vi "IMMU - Standalone Main.vi"() -> ()   [LabVIEW 2021]
uses:
  Lab 5/Lab 5 Code/Heading_TDef.ctl
  <vilib>/Platform/TimedLoop/XDataNode/timing_clust.ctl
  <vilib>/Platform/TimedLoop/XDataNode/nitl_modes.ctl
  <vilib>/Platform/TimedLoop/XDataNode/wakeup.ctl
  <vilib>/platform/TimedLoop/XDataNode/XDataNode.xnode
  <vilib>/myRIO/Express VI/Onboard IO/I2C/I2C Express VI.xnode
  <vilib>/myRIO/Instrument Drivers/Onboard IO/I2C/vis/Configure.vi
  <vilib>/myRIO/Instrument Drivers/Onboard IO/I2C/I2C.lvlib
  <vilib>/myRIO/Instrument Drivers/Onboard IO/I2C/typedefs/I2C Transfer Rate.ctl
  <vilib>/myRIO/Instrument Drivers/Onboard IO/I2C/typedefs/I2C User Configuration.ctl
  <vilib>/myRIO/Instrument Drivers/Onboard IO/I2C/typedefs/I2C Configuration.ctl
  <vilib>/myRIO/Common/Instrument Driver Framework/myRIO v1.0/I2C/typedefs/I2C Channels Enum.ctl
  <vilib>/myRIO/Common/Instrument Driver Framework/Utilities/typedefs/Generic FPGA Reference.ctl
  <vilib>/myRIO/Common/Instrument Driver Framework/Utilities/typedefs/myRIO v1.0 Reference.ctl
  <vilib>/myRIO/Common/Instrument Driver Framework/Utilities/typedefs/Hardware Version Enum.ctl
  <vilib>/myRIO/Common/Instrument Driver Framework/Utilities/typedefs/myRIO Generic Hardware Reference.ctl
  <vilib>/myRIO/Instrument Drivers/Onboard IO/I2C/typedefs/I2C Reference.ctl
  <vilib>/myRIO/Instrument Drivers/Onboard IO/I2C/vis/myRIO I2C Open.xnode
  <vilib>/myRIO/Common/Instrument Driver Framework/Utilities/vis/Is FPGA Ref Available.vi
  <vilib>/myRIO/Common/Instrument Driver Framework/myRIO v1.0/I2C/vis/myRIO v1.1 Open I2C.vi
  <vilib>/userDefined/High Color/nirio_resource_hc.ctl
  <vilib>/myRIO/Instrument Drivers/Onboard IO/I2C/vis/Write.vi
  <vilib>/Platform/TimedLoop/XDataNode/XDNodeRunTimeDep.lvlib
panel:
  out "Output Offset Array (int)":i16[](array[numeric])
  out "Mag Flux (uT)":T1(graph)
  out "Heading Output (Str)":T2
  out "Heading":dbl
  in  "Reset Gyro":bool
  out "Acceleration (g)":T3(graph)
  out "Velocity":T1(graph)
  out "Rotation":T3(graph)
  out "Acceleration (ms^2)":dbl[](array[numeric])
  out "error out":errorcluster
  out "Velocity Cluster Out":cluster{i16, i16, i16}
  out "Rotation Cluster Out":T4
  in  "stop":bool
  in  "error in (no error)":errorcluster
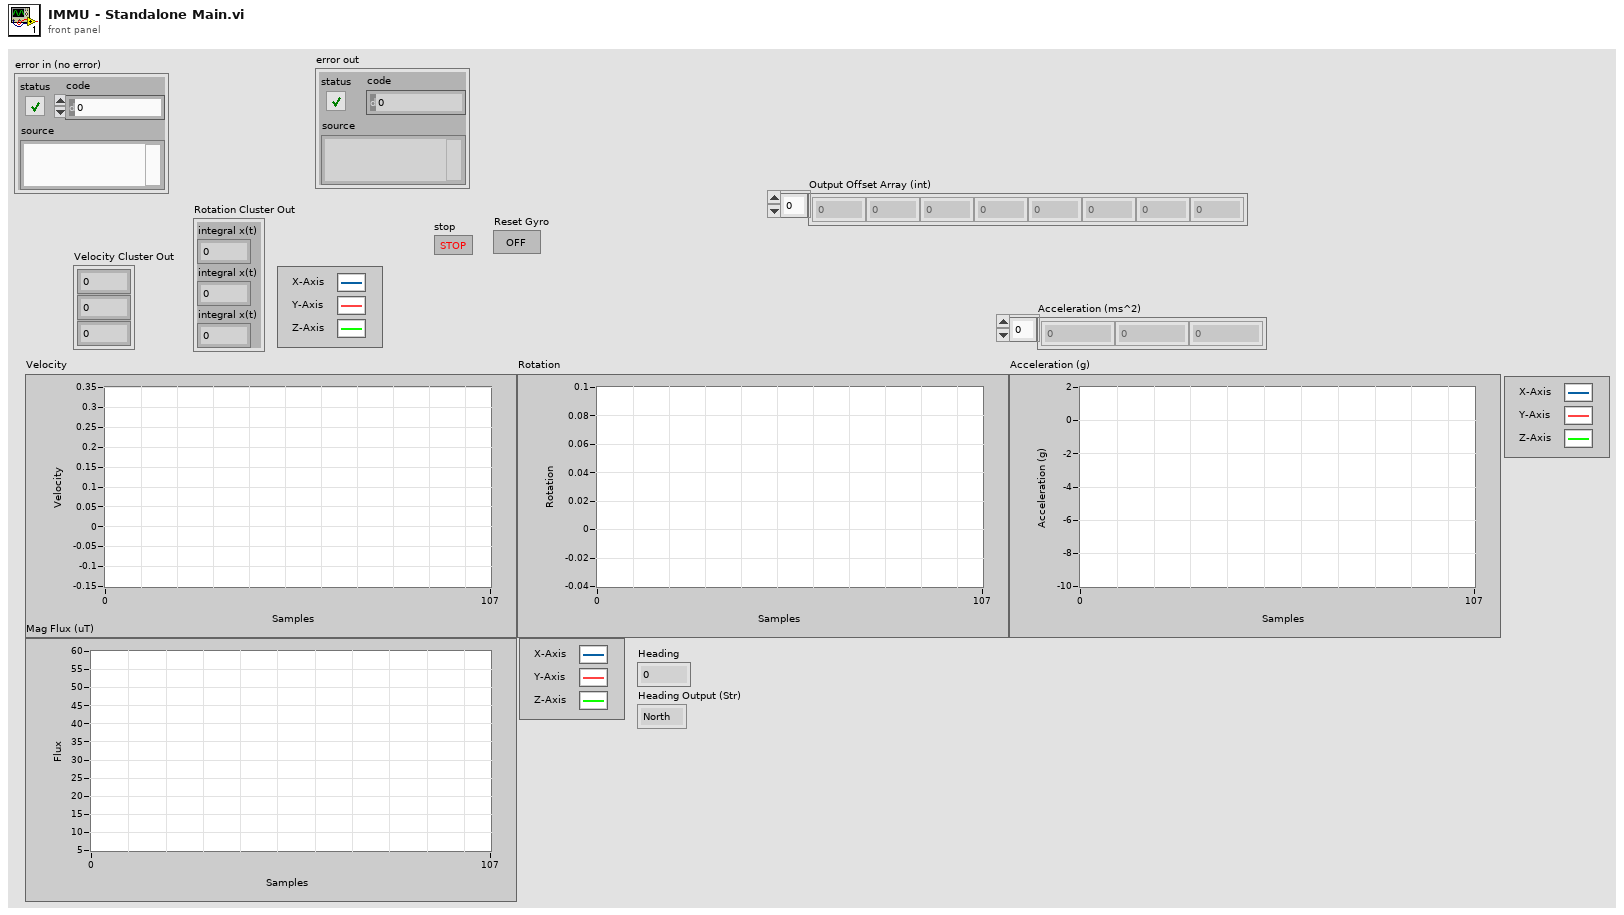
[diagram p1: front panel]
types:
  T1 = cluster{"Velocity":dbl, "Velocity":dbl, "Velocity":dbl}
  T2 = typedef "Heading_TDef.ctl" = enum16{"North ", "North East", "East", "Southeast", "South", "Southwest", "West", "Northwest"}
  T3 = cluster{"X-Axis":dbl, "Y-Axis":dbl, "Z-Axis":dbl}
  T4 = cluster{"integral x(t)":dbl, "integral x(t)":dbl, "integral x(t)":dbl}
  T5 = typedef "I2C.lvlib/I2C Reference.ctl" = cluster{"myRIO Reference":T6, "I2C Channels Enum":T10, "I2C Configuration":T11}
  T6 = typedef "myRIO Generic Hardware Reference.ctl" = cluster{"myRIO Model":T7, "myRIO Hardware Reference":T8}
  T7 = typedef "Hardware Version Enum.ctl" = enum16{"Unknown", "myRIO-1900", "myRIO-1950", "roboRIO", "NI ELVIS RIO CM", "ELVIS III"}
  T8 = typedef "myRIO v1.0 Reference.ctl" = cluster{"Generic FPGA Reference":T9, "Allow multiple opens":bool}
  T9 = typedef "Generic FPGA Reference.ctl" = refnum<k20>
  T10 = typedef "I2C Channels Enum.ctl" = enum16{"Not Connected", "A/I2C", "B/I2C", "I2C/I2C"}
  T11 = typedef "I2C.lvlib/I2C Configuration.ctl" = cluster{"I2C Transfer Rate":T12}
  T12 = typedef "I2C.lvlib/I2C Transfer Rate.ctl" = enum16{"Standard mode (100 kbps)", "Fast mode (400 kbps)"}
  T13 = typedef "I2C.lvlib/I2C User Configuration.ctl" = cluster{"I2C Transfer Rate":T12}
  T14 = typedef "nirio_resource_hc.ctl" = tag
  T15 = typedef "XDNodeRunTimeDep.lvlib/timing_clust.ctl" = cluster{"Expected End [f-1]":u64, "Actual End [f-1]":u64, "Finished Late? [f-1]":bool, "Expected End [i-1]":u64, "Actual End [i-1]":u64, "Finished Late? [i-1]":bool, "Expected Start [i]":u64, "Actual Start [i]":u64, "Expected Start [f]":u64, "Actual Start [f]":u64, "Source Name":string, "Structure Name":string, "Period":i64, "Deadline":i64, "Offset":i64, "Start":i64, "Priority":i32, "Timeout":i32, "Mode":T16, "Wakeup Reason":T17, "Error":errorcluster, "Source Type":string, "Secondary Source Type":string, "Global End Time":u64, "Global Start Time":u64, "Frame Duration":u64, "Iteration Duration":u64, "Assigned CPU":i32, "I/O Scan Engine Mode":u32}
  T16 = typedef "XDNodeRunTimeDep.lvlib/nitl_modes.ctl" = enum32{"No Change", "Process missed periods, maintain original phase", "Discard missed periods, maintain original phase", "Process missed periods, ignore original phase", "Discard missed periods, ignore original phase"}
  T17 = typedef "XDNodeRunTimeDep.lvlib/wakeup.ctl" = enum32{"Normal", "Aborted", "Asynchronous wakeup", "Timing source error", "Timed loop error", "Timeout"}
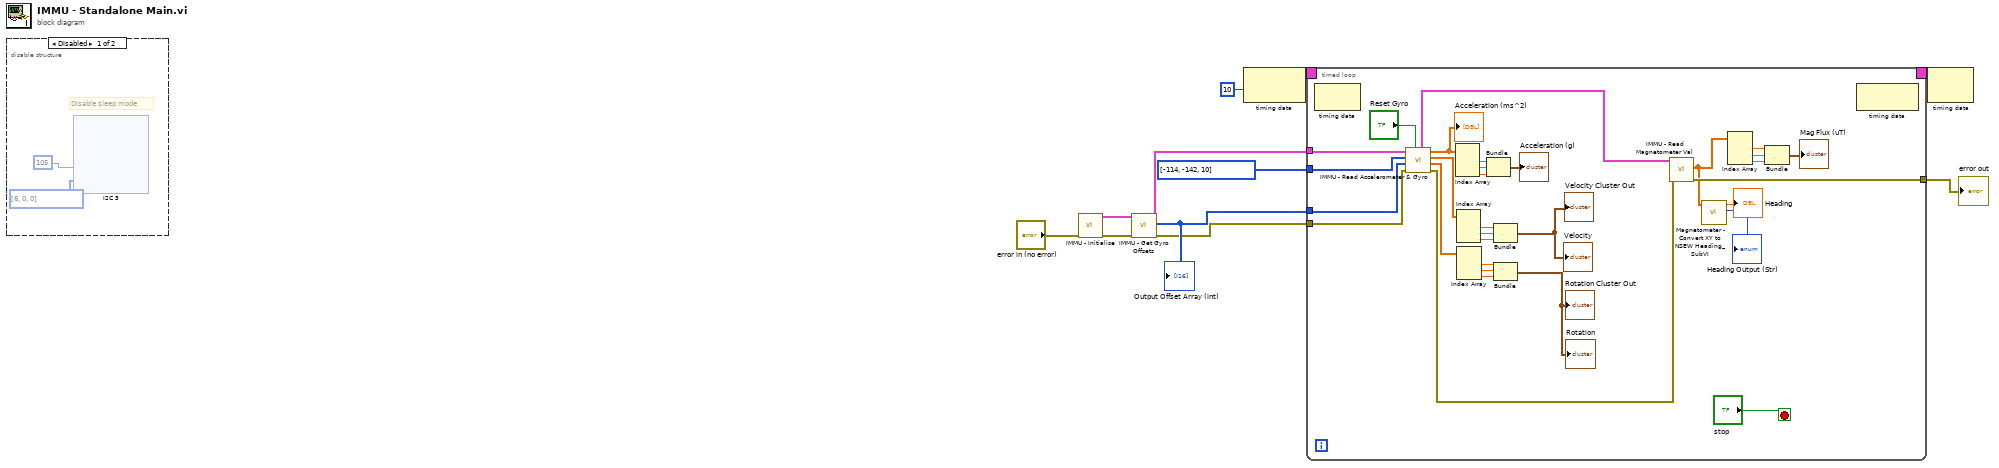
[diagram p0: block diagram]
diagram:
  n1 = disable-structure shown="Disabled" {
    frame Disabled {
      # "Disable sleep mode"
      n2 = xnode "I2C 3"("Slave Address (7-bit)"=u8 105, "Bytes to Write"=u8[] [6, 0, 0]) -> ()  [unwired: 1 in, 1 out]
    }
    frame Enabled {
    }
  }
  n3 = call "IMMU - Initialise.vi"("error in (no error)"="error in (no error)") -> ("error out"=w7:errorcluster, "I2C Ref Out"=w6:T5)  [unwired: 9 in]
  n4 = call "IMMU - Get Gyro Offsets.vi"("error in (no error)"=w7, "I2C Ref In"=w6) -> ("error out"=w2:errorcluster, "Output Offset Array (int)"=w5:i16[], "I2C Ref Out"=w3:T5)  [unwired: 7 in]
  "Output Offset Array (int)" <- w5
  n5 = node-c288(i64 10 ("Period")) -> (w11:T15)
  n6 = timed-loop {
    timing: w11 -> [_]
    timing-out: [_] -> w10
    tunnel: w3 -> [w69]
    tunnel: w2 -> [w68]
    tunnel: w5 -> [w53]
    tunnel: [w60] -> w4
    tunnel: i16[] [-114, -142, 10] ("Accel Offset Array In") -> [w52]
    stop <- "stop" stop-if-true
    n7 = node-c288() -> ()  [unwired: 1 in, 1 out]
    n8 = call "IMMU - Read Accelerometer & Gyro.vi"("Reset Gyro"="Reset Gyro", "error in (no error)"=w68, "Gyro Offset Array In"=w53, "Accel Offset Array In"=w52, "I2C Ref In"=w69) -> ("error out"=w63:errorcluster, "Gyro Rotation Out (degrees)"=w65:dbl[], "Gyro Rotational Velocity Out (deg/s)"=w66:dbl[], "Output Acceleration Array (ms^2)"=w64:dbl[], "I2C Ref Out"=w59:T5)  [unwired: 2 in]
    "Acceleration (ms^2)" <- w64
    n9 = Index Array(array=w64) -> (element #1=w81:dbl, element #2=w80:dbl, element #3=w79:dbl)  [unwired: 3 in]
    n10 = Index Array(array=w66) -> (element #1=w77:dbl, element #2=w76:dbl, element #3=w75:dbl)  [unwired: 3 in]
    n11 = Index Array(array=w65) -> (element #1=w74:dbl, element #2=w73:dbl, element #3=w72:dbl)  [unwired: 3 in]
    n12 = Bundle(w81, w80, w79) -> (→"Acceleration (g)":cluster{dbl, dbl, dbl})  [unwired: 1 in]
    n13 = Bundle(w77, w76, w75) -> (→"Velocity Cluster Out" →"Velocity":cluster{dbl, dbl, dbl})  [unwired: 1 in]
    n14 = Bundle("integral x(t)"=w74, "integral x(t)"=w73, "integral x(t)"=w72) -> (→"Rotation Cluster Out" →"Rotation":T4)  [unwired: 1 in]
    n15 = call "IMMU - Read Magnetometer Val.vi"("error in (no error)"=w63, "I2C Ref In"=w59) -> ("error out"=w60:errorcluster, "Magnetometer Flux Out (uT)"=w56:dbl[])  [unwired: 7 in, 1 out]
    n16 = call "Magnetometer - Convert XY to NSEW Heading_SubVI.vi"("Flux In (uT)"=w56) -> ("Heading Output (Str)"=→"Heading Output (Str)":T2, "Heading"=→"Heading":dbl)  [unwired: 9 in]
    n17 = Index Array(array=w56) -> (element #1=w58:dbl, element #2=w57:dbl, element #3=w55:dbl)  [unwired: 3 in]
    n18 = Bundle(w58, w57, w55) -> (→"Mag Flux (uT)":cluster{dbl, dbl, dbl})  [unwired: 1 in]
    n19 = node-c288() -> ()  [unwired: 1 in, 1 out]
  }
  "error out" <- w4
  n20 = node-c288(w10) -> ()  [unwired: 1 out]
